vi "RT test.vi"() -> ()   [LabVIEW 2014]
uses:
  <vilib>/Platform/TimedLoop/XDataNode/timing_clust.ctl
  <vilib>/Platform/TimedLoop/XDataNode/nitl_modes.ctl
  <vilib>/Platform/TimedLoop/XDataNode/wakeup.ctl
  <vilib>/Analysis/3filter.llb/Filter Passband Type.ctl
  <vilib>/FPGAPlugInAG/cRIO-9066/niLvFpga_Open_cRIO-9066.vi
  <vilib>/rvi/interface/common/dynamic/niFpgaDynamicAddResources.vi
  <vilib>/ethernetip/ethernetip.llb/EthernetIP Tag Write Raw.vi
  <vilib>/ethernetip/ethernetip.llb/EthernetIP Tag Write REAL.vi
  <vilib>/ethernetip/ethernetip.llb/EthernetIP Tag Write BOOL.vi
  <vilib>/Utility/error.llb/Error Cluster From Error Code.vi
  <vilib>/rvi/errors/niLvFpgaAdjustHostInterfaceError.vi
  <vilib>/Platform/TimedLoop/XDataNode/XDataNode.xnode
  <vilib>/rvi/interface/nirviOpenFPGA/nirviOpenFPGA.xnode
  FPGA Bitfiles/SMSLDrill_FPGATarget_SMSL-DrillFPGA_76AJMwWUk6w.lvbitx
  FPGA/SMSL-Drill FPGA.vi
  <vilib>/rvi/interface/nirviReadWriteControl/nirviReadWriteControl.xnode
  <vilib>/Platform/TimedLoop/XDataNode/XDNodeRunTimeDep.lvlib
  <vilib>/NI_Real-Time Target Support.lvlib
  NiFpgaLv.dll
  <vilib>/rvi/interface/Simulation/niFpgaSimulationCallBeginRW.vi
  <vilib>/ptbypt/NI_PtbyPt.lvlib
  <vilib>/Analysis/NI_AALBase.lvlib
  <vilib>/ethernetip/ethernetip.lvlib
panel:
  in  "advance file":bool
  in  "Log":bool
  in  "Data 2":bool[](array[boolean])=[FALSE, FALSE, FALSE, FALSE, FALSE, FALSE, FALSE, FALSE, FALSE, FALSE, FALSE, FALSE, FALSE, FALSE, FALSE, FALSE, FALSE, FALSE, FALSE, FALSE, FALSE, FALSE, FALSE, FALSE, FALSE, FALSE, FALSE, FALSE, FALSE, FALSE]
  in  "Reverse       Forward":bool
  in  "Data":bool[](array[boolean])=[FALSE, FALSE, FALSE, FALSE, FALSE, FALSE, FALSE, FALSE, FALSE, FALSE, FALSE, FALSE, FALSE, FALSE, FALSE, FALSE, FALSE, FALSE, FALSE, FALSE, FALSE, FALSE, FALSE, FALSE, FALSE, FALSE, FALSE, FALSE, FALSE]
  in  "Timeout (ms)":i32=1000
  in  "Move":bool
  in  "RPM":dbl
  in  "ACC":dbl=1.0
  in  "DEC":dbl=1.0
  in  "JERK":dbl=1.0
  in  "Enable Rotary":bool
  in  "Enable/Disable":bool
  in  "Speed Command [Inch/S]":dbl
  in  "Inch / Step":dbl=0.003
  in  "Manual":bool
  in  "Frequency [Hz]":dbl
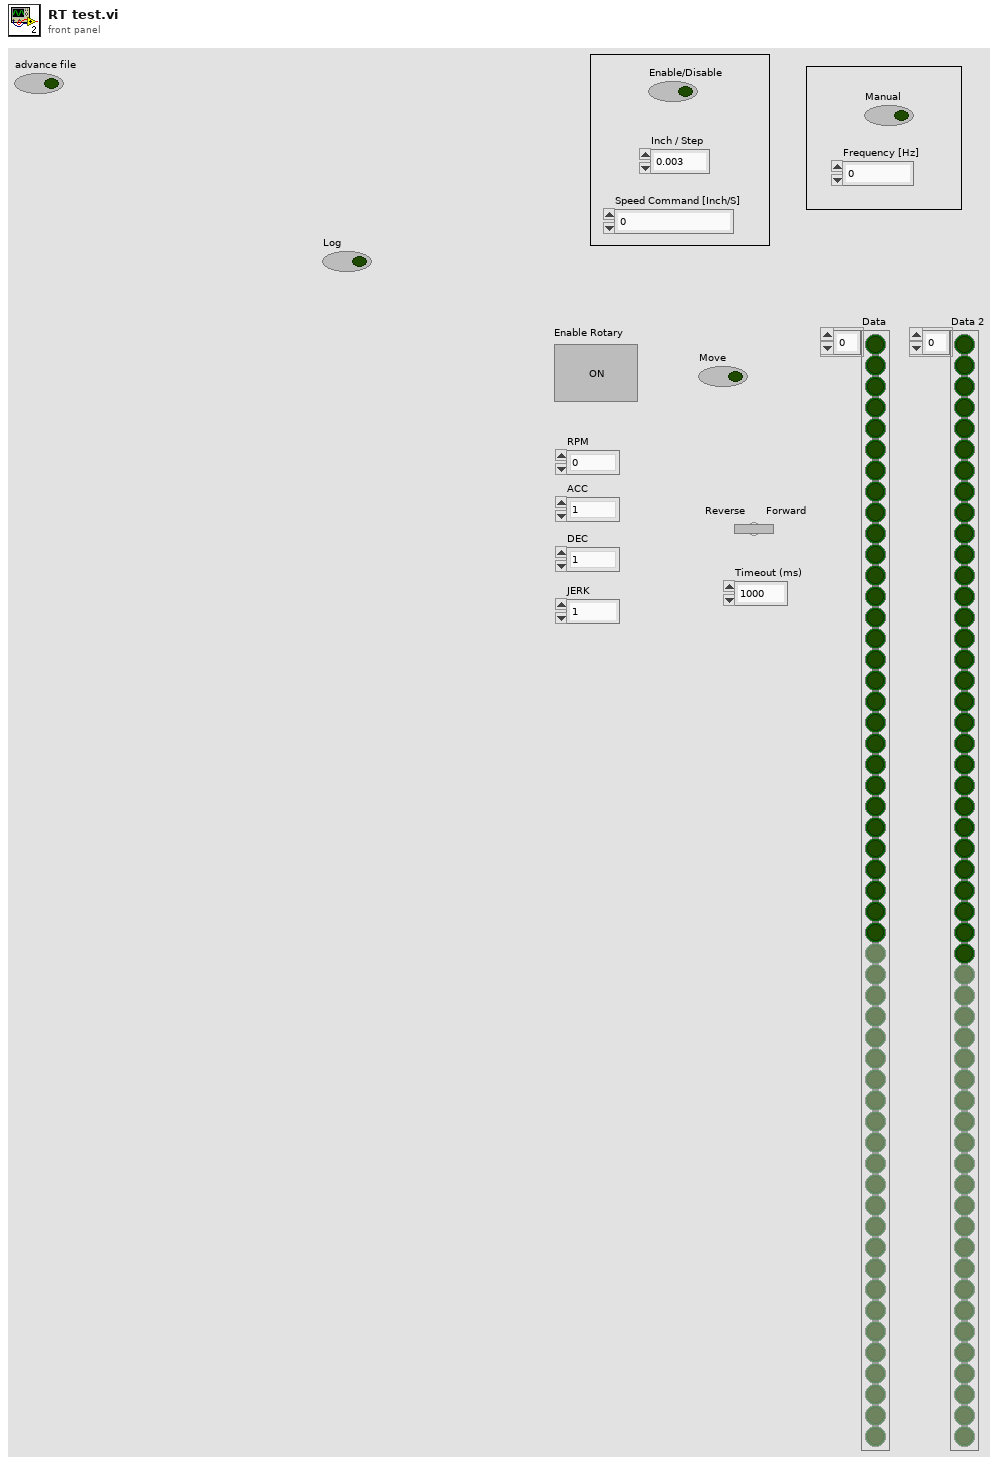
[diagram p1: front panel]
types:
  T1 = enum16{"open", "open or create", "create or replace", "create", "open (read only)"}
  T2 = typedef "XDNodeRunTimeDep.lvlib/timing_clust.ctl" = cluster{"Expected End [f-1]":u64, "Actual End [f-1]":u64, "Finished Late? [f-1]":bool, "Expected End [i-1]":u64, "Actual End [i-1]":u64, "Finished Late? [i-1]":bool, "Expected Start [i]":u64, "Actual Start [i]":u64, "Expected Start [f]":u64, "Actual Start [f]":u64, "Source Name":string, "Structure Name":string, "Period":i64, "Deadline":i64, "Offset":i64, "Start":i64, "Priority":i32, "Timeout":i32, "Mode":T3, "Wakeup Reason":T4, "Error":errorcluster, "Source Type":string, "Secondary Source Type":string, "Global End Time":u64, "Global Start Time":u64, "Frame Duration":u64, "Iteration Duration":u64, "Assigned CPU":i32, "I/O Scan Engine Mode":u32}
  T3 = typedef "XDNodeRunTimeDep.lvlib/nitl_modes.ctl" = enum32{"No Change", "Process missed periods, maintain original phase", "Discard missed periods, maintain original phase", "Process missed periods, ignore original phase", "Discard missed periods, ignore original phase"}
  T4 = typedef "XDNodeRunTimeDep.lvlib/wakeup.ctl" = enum32{"Normal", "Aborted", "Asynchronous wakeup", "Timing source error", "Timed loop error", "Timeout"}
  T5 = typedef "NI_AALBase.lvlib/Filter Passband Type.ctl" = enum32{"Lowpass", "Highpass", "Bandpass", "Bandstop"}
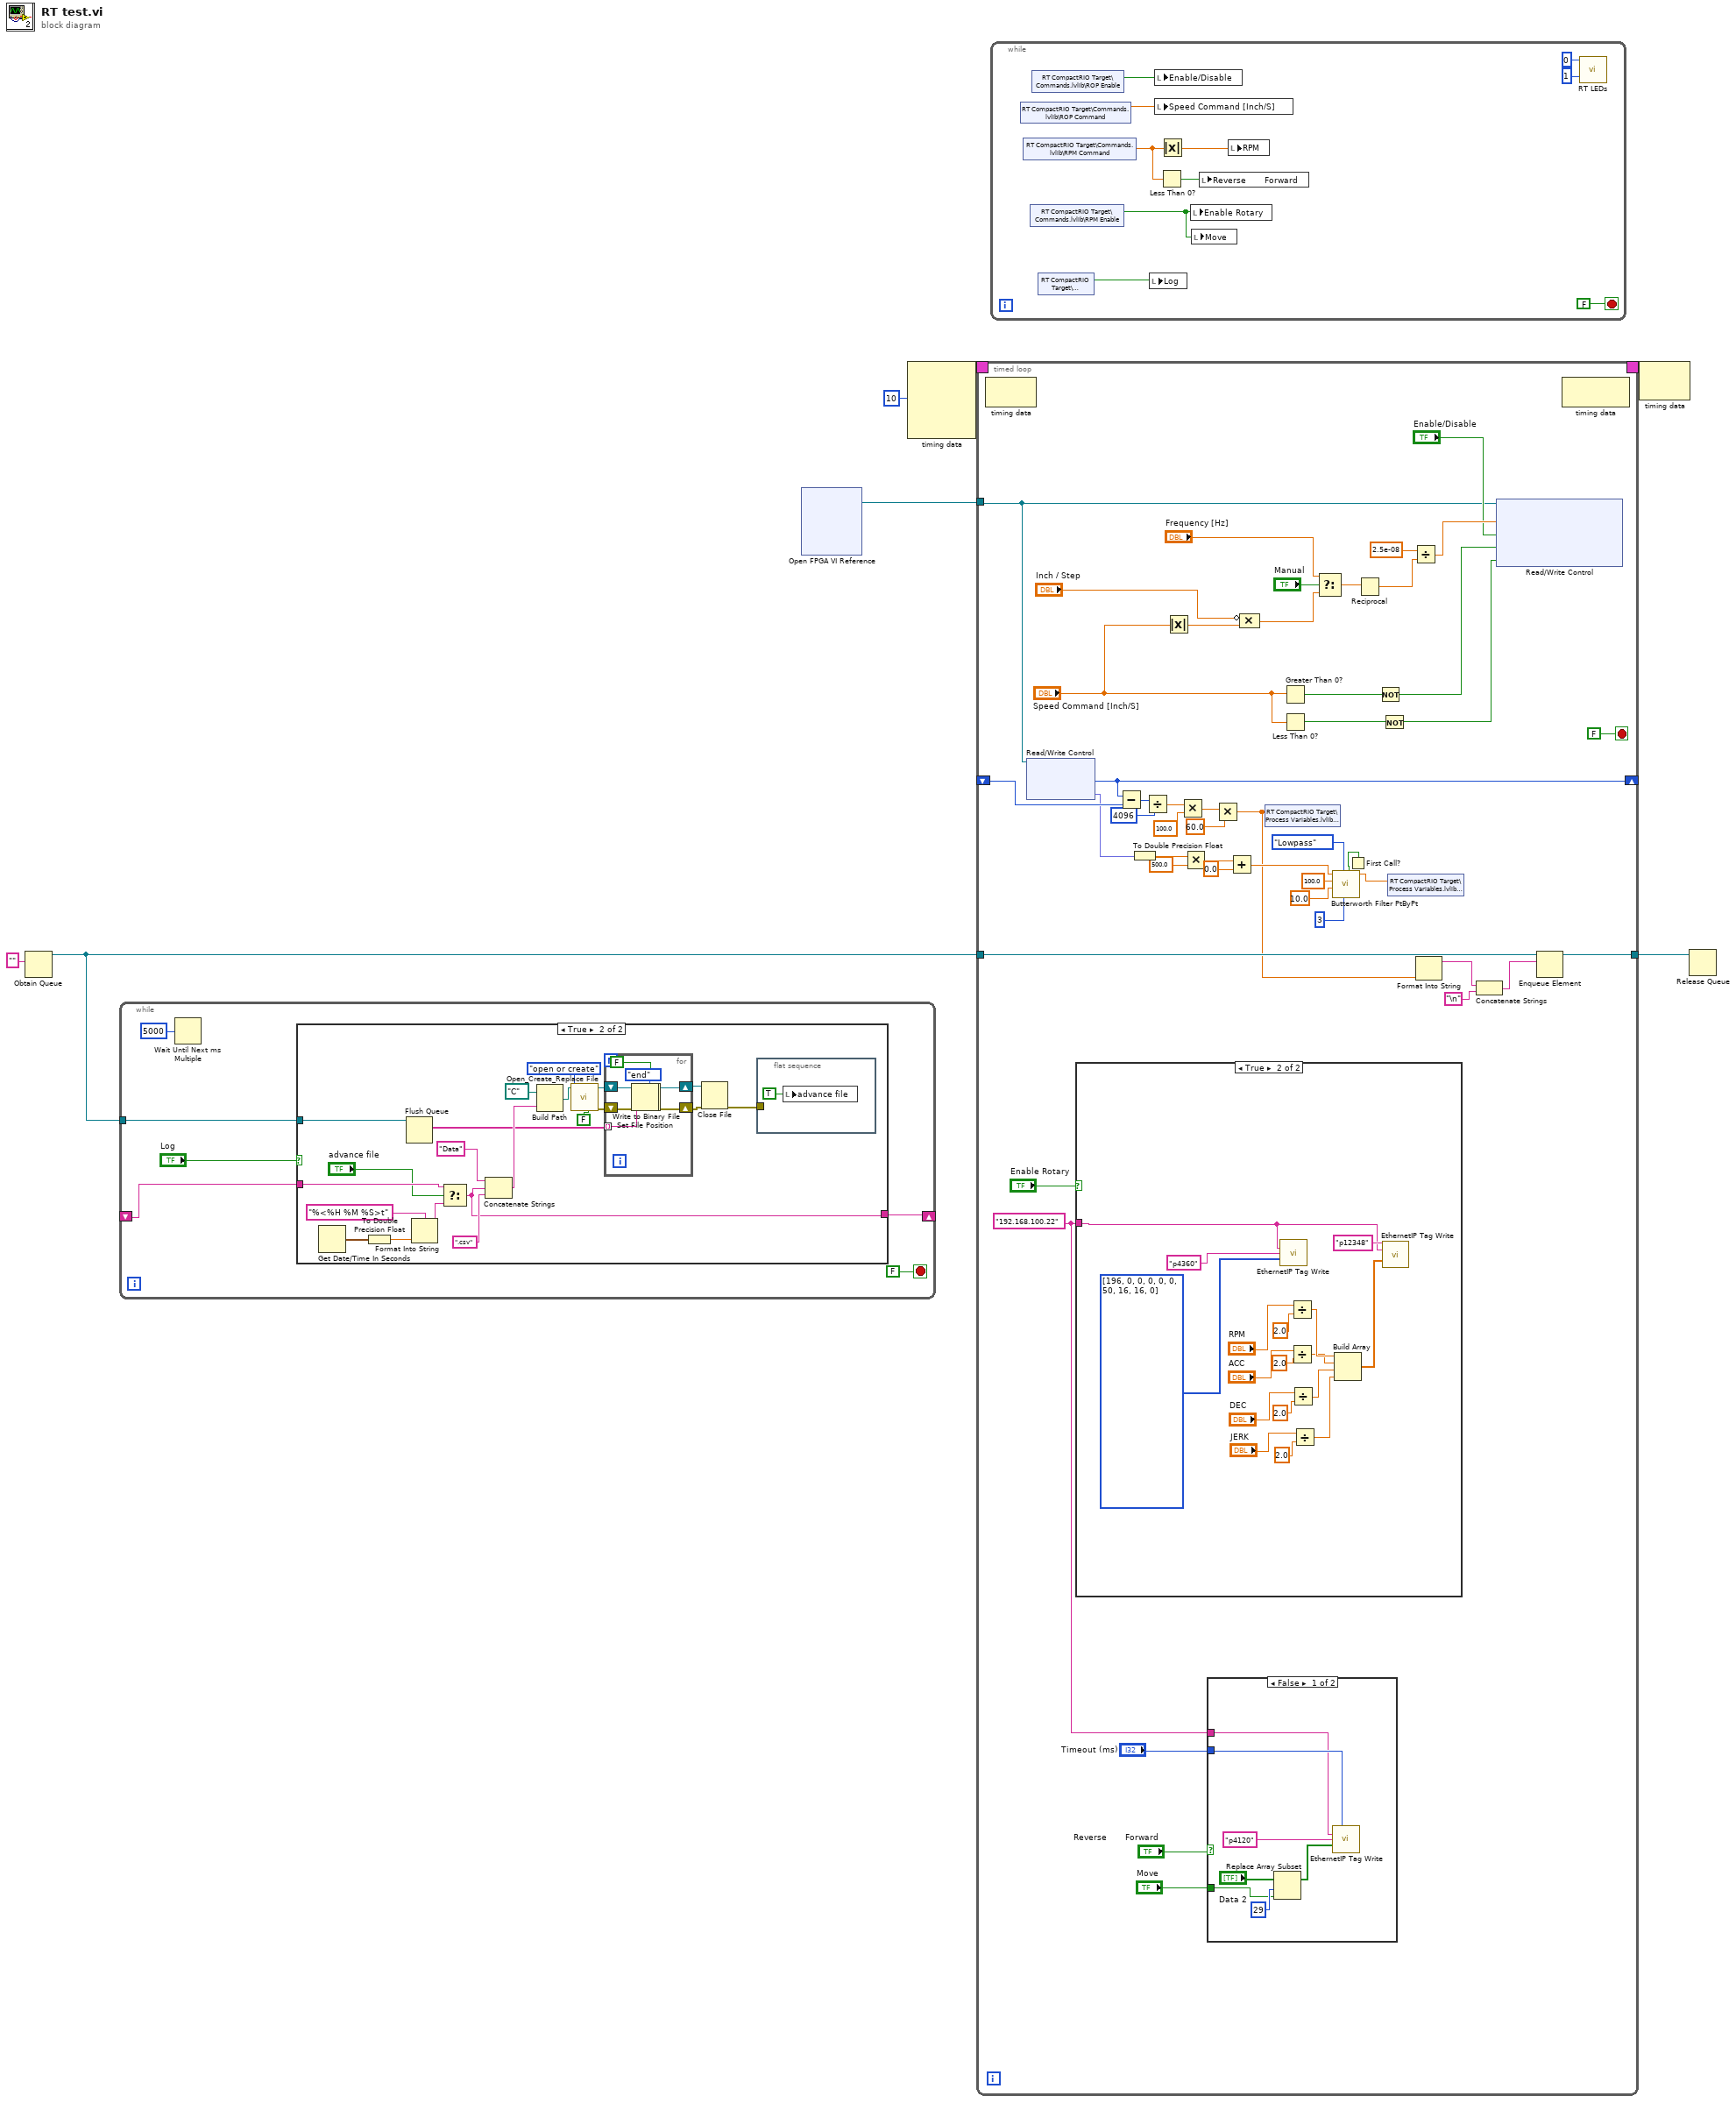
[diagram p0: block diagram]
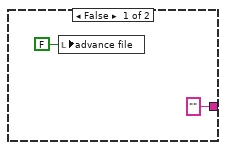
[diagram p2: hidden frame]
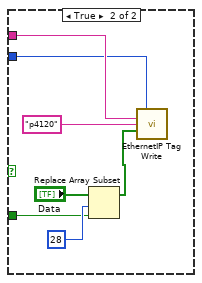
[diagram p3: hidden frame]
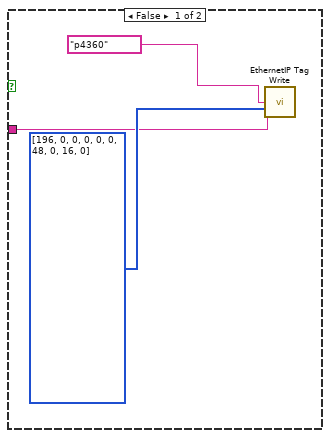
[diagram p4: hidden frame]
diagram:
  n1 = Obtain Queue(element data type="" ("initial string")) -> (queue out=w1:refnum<queue>)  [unwired: 4 in, 2 out]
  n2 = while {
    tunnel: w1 -> [w12]
    shift-right: [w9] -> _
    shift-left: _ -> [w8]
    stop <- FALSE stop-if-true
    n3 = Wait Until Next ms Multiple(millisecond multiple=u32 5000) -> ()  [unwired: 1 out]
    n4 = case shown="True" "Log" {
      tunnel: w12 -> [_ w36]
      tunnel: ["" w16] -> w9
      tunnel: w8 -> [_ w20]
      frame False {
        n5 = local write "advance file"(FALSE ("advance file")) -> ()
      }
      frame True {
        n6 = Get Date/Time In Seconds() -> (seconds since 1Jan1904=w21:timestamp)
        n7 = To Double Precision Float(number=w21) -> (double precision float=w22:dbl)
        n8 = Flush Queue(queue=w36) -> (remaining elements=w27:string[])  [unwired: 1 in, 2 out]
        n9 = Format Into String(format string="%<%H %M %S>t", w22) -> (resulting string=w17:string)  [unwired: 2 in, 1 out]
        n10 = Select(t=w20, s="advance file", f=w17) -> (s? t:f=w16:string)
        n11 = Concatenate Strings("Data" ("string"), w16, ".csv") -> (w28:string)
        n12 = Build Path(base path=path "C:/", name or relative path=w28) -> (appended path=w29:path)
        n13 = call <vilib>:"Open_Create_Replace File.vi"("advisory dialog? (display:T)"=FALSE, "function (open:0)"=T1."open or create", "file path"=w29) -> ("error out"=w32:errorcluster, "refnum"=w33:refnum<file>)  [unwired: 5 in, 2 out]
        n14 = for {
          shift-right: [w42] -> w31
          shift-left: w33 -> [w46]
          shift-right: [w43] -> w30
          shift-left: w32 -> [w44]
          tunnel: w27 -> [w41] mode=indexing
          n15 = Set File Position(refnum=w46, from (0:start)=enum16{"start", "end", "current"}."end" ("pos mode (0:2)"), error in=w44) -> (refnum out=w40:refnum<file>, error out=w39:errorcluster)  [unwired: 1 in]
          n16 = Write to Binary File(file (use dialog)=w40, data=w41, error in=w39, 5:FALSE ("prepend array or string size? (T)")) -> (refnum out=w42:refnum<file>, error out=w43:errorcluster)  [unwired: 2 in, 1 out]
        }
        n17 = Close File(refnum=w31, error in=w30) -> (error out=w18:errorcluster)  [unwired: 1 out]
        n18 = flat-sequence {
          tunnel: w18 -> [_]
          frame #0 {
            n19 = local write "advance file"(TRUE ("advance file")) -> ()
          }
        }
      }
    }
  }
  n20 = xnode "Open FPGA VI Reference"() -> ("FPGA VI Reference Out"=w5:refnum<k20>)  [unwired: 2 in, 1 out]
  n21 = node-c288(i64 10 ("Period")) -> (w7:T2)  [unwired: 3 in]
  n22 = timed-loop {
    timing: w7 -> [_]
    timing-out: [_] -> w6
    tunnel: w5 -> [w78]
    shift-right: [w77] -> _
    shift-left: _ -> [w76]
    tunnel: w1 -> [w52]
    tunnel: [w50] -> w2
    stop <- FALSE stop-if-true
    w53 = "192.168.100.22" ("Network Path")
    n23 = node-c288() -> ()  [unwired: 1 in, 1 out]
    n24 = xnode "Read/Write Control"("FPGA VI Reference In"=w78) -> ("Bit Position"=w77:i32, "Mod2/AI0"=w69:fxp<+/-,24,5>)  [unwired: 1 in, 2 out]
    n25 = case shown="True" "Enable Rotary" {
      tunnel: w53 -> [w109 w124]
      frame False {
        n26 = call-poly <vilib>:"EthernetIP Tag Write.vi"("Network Path"=w109, "Tag Name"="p4360", "Data"=u8[] [196, 0, 0, 0, 0, 0, 48, 0, 16, 0]) -> ()  [unwired: 11 in, 2 out]
      }
      frame True {
        n27 = call-poly <vilib>:"EthernetIP Tag Write.vi"("Network Path"=w124, "Tag Name"="p4360", "Data"=u8[] [196, 0, 0, 0, 0, 0, 50, 16, 16, 0]) -> ()  [unwired: 11 in, 2 out]
        n28 = Divide(x="RPM", y=2.0) -> (x/y=w121:dbl)
        n29 = Divide(x="ACC", y=2.0) -> (x/y=w114:dbl)
        n30 = Divide(x="DEC", y=2.0) -> (x/y=w112:dbl)
        n31 = Divide(x="JERK", y=2.0) -> (x/y=w113:dbl)
        n32 = Build Array(w121, w114, w112, w113) -> (w126:dbl[])
        n33 = call-poly <vilib>:"EthernetIP Tag Write.vi"("Network Path"=w124, "Tag Name"="p12348", "Data"=w126) -> ()  [unwired: 11 in, 2 out]
      }
    }
    n34 = Subtract(x=w77, y=w76) -> (x-y=w75:i32)
    n35 = To Double Precision Float(number=w69) -> (double precision float=w67:dbl)
    n36 = Divide(x=w75, y=4096) -> (x/y=w73:dbl)
    n37 = Absolute Value(x="Speed Command [Inch/S]") -> (abs(x)=w83:dbl)
    n38 = Multiply(x=w73, y=100.0) -> (x*y=w72:dbl)
    n39 = Multiply(x=w67, y=500.0) -> (x*y=w68:dbl)
    n40 = case shown="False" "Reverse       Forward" {
      tunnel: "Move" -> [w100 w107]
      tunnel: w53 -> [w96 w104]
      tunnel: "Timeout (ms)" -> [w97 w103]
      frame False {
        n41 = Replace Array Subset(array="Data 2", new element=w100, index=29) -> (w99:bool[])
        n42 = call-poly <vilib>:"EthernetIP Tag Write.vi"("Timeout (ms)"=w97, "Network Path"=w96, "Tag Name"="p4120" ("Tag Name 2"), "Data"=w99) -> ()  [unwired: 10 in, 2 out]
      }
      frame True {
        n43 = Replace Array Subset(array="Data", new element=w107, index=28) -> (w106:bool[])
        n44 = call-poly <vilib>:"EthernetIP Tag Write.vi"("Timeout (ms)"=w103, "Network Path"=w104, "Tag Name"="p4120", "Data"=w106) -> ()  [unwired: 10 in, 2 out]
      }
    }
    n45 = Multiply(x=w72, y=60.0) -> (x*y=w51:dbl)
    n46 = Add(x=w68, y=0.0) -> (x+y=w61:dbl)
    n47 = Compound Arithmetic op=MULTIPLY(invert "Inch / Step", w83) -> (w88:dbl)
    n48 = shared-variable "RT CompactRIO Target\\Process Variables.lvlib\\Bit RPM"(w51) -> ()  [unwired: 1 in, 1 out]
    n49 = Greater Than 0?(x="Speed Command [Inch/S]") -> (x > 0?=w84:bool)
    n50 = Less Than 0?(x="Speed Command [Inch/S]") -> (x < 0?=w81:bool)
    n51 = Select(t="Frequency [Hz]", s="Manual", f=w88) -> (s? t:f=w91:dbl)
    n52 = First Call?() -> (First Call?: T/F=w62:bool)
    n53 = call <vilib>:"Butterworth Filter PtByPt.vi"("initialize"=w62, "order"=3, "filter type"=Filter_Passband_Type."Lowpass", "high cutoff freq: fh"=10.0 ("low cutoff freq: fl"), "sampling freq: fs"=100.0, "x"=w61) -> ("Filtered x"=w64:dbl)  [unwired: 3 in, 1 out]
    n54 = Reciprocal(x=w91) -> (1/x=w92:dbl)
    n55 = Not(x=w84) -> (.not. x?=w80:bool)
    n56 = Not(x=w81) -> (.not. x?=w79:bool)
    n57 = shared-variable "RT CompactRIO Target\\Process Variables.lvlib\\Bit Load"(w64) -> ()  [unwired: 1 in, 1 out]
    n58 = Divide(x=2.5e-08 ("y"), y=w92) -> (x/y=w93:dbl)
    n59 = Format Into String(w51) -> (resulting string=w49:string)  [unwired: 3 in, 1 out]
    n60 = Concatenate Strings(w49, "\n") -> (w48:string)
    n61 = xnode "Read/Write Control"("FPGA VI Reference In"=w78, "frequency (periods/tick)"=w93, "Enable/Disable"="Enable/Disable", "Direction FWD"=w80, "Direction BKWD"=w79) -> ()  [unwired: 1 in, 2 out]
    n62 = Enqueue Element(queue=w52, element=w48) -> (queue out=w50:refnum<queue>)  [unwired: 2 in, 2 out]
    n63 = node-c288() -> ()  [unwired: 1 in, 1 out]
  }
  n64 = while {
    stop <- FALSE stop-if-true
    n65 = shared-variable "RT CompactRIO Target\\Commands.lvlib\\ROP Command"() -> (w138:dbl)  [unwired: 1 in, 1 out]
    n66 = shared-variable "RT CompactRIO Target\\Commands.lvlib\\RPM Command"() -> (w133:dbl)  [unwired: 1 in, 1 out]
    n67 = shared-variable "RT CompactRIO Target\\Commands.lvlib\\RPM Enable"() -> (w135:bool)  [unwired: 1 in, 1 out]
    n68 = shared-variable "RT CompactRIO Target\\Commands.lvlib\\ROP Enable"() -> (w139:bool)  [unwired: 1 in, 1 out]
    n69 = shared-variable "RT CompactRIO Target\\Commands.lvlib\\Log"() -> (w131:bool)  [unwired: 1 in, 1 out]
    n70 = local write "Log"(w131) -> ()
    n71 = local write "Enable/Disable"(w139) -> ()
    n72 = local write "Speed Command [Inch/S]"(w138) -> ()
    n73 = Less Than 0?(x=w133) -> (x < 0?=w134:bool)
    n74 = Absolute Value(x=w133) -> (abs(x)=w132:dbl)
    n75 = local write "Enable Rotary"(w135) -> ()
    n76 = local write "Move"(w135) -> ()
    n77 = local write "Reverse       Forward"(w134) -> ()
    n78 = local write "RPM"(w132) -> ()
    n79 = call <vilib>:"RT LEDs.vi"("State"=1, "LED Num"=0) -> ()  [unwired: 4 in, 2 out]
  }
  n80 = node-c288(w6) -> ()  [unwired: 1 out]
  n81 = Release Queue(queue=w2) -> ()  [unwired: 2 in, 3 out]
